vi "Do3.vi"(8 "error in (no error)":errorcluster, 11 "object in":refnum<class "Sub.lvclass">) -> (0 "error out":errorcluster, 2 "Numeric":i32, 3 "object out":refnum<class "Sub.lvclass">)   [LabVIEW 2019, in "Sub.lvclass"]
uses:
  Sub.lvclass
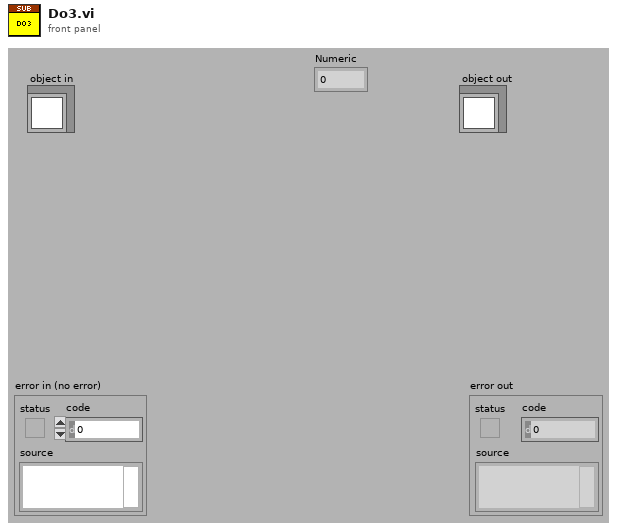
[diagram p1: front panel]
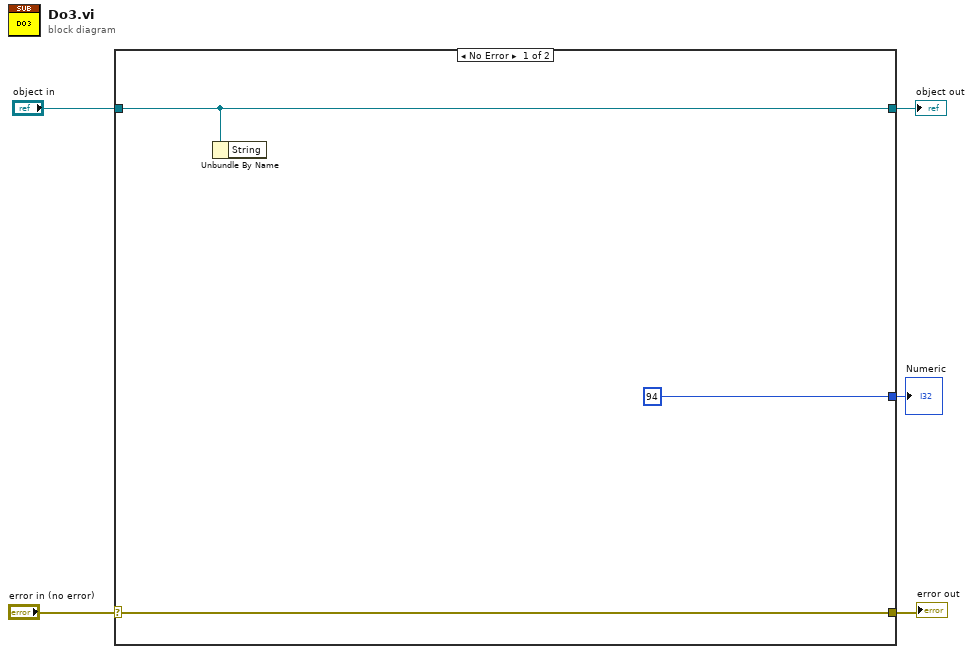
[diagram p0: block diagram]
diagram:
  n1 = case shown="No Error" "error in (no error)" {
    selector: "error in (no error)" -> [w8 w10]
    tunnel: [w8 w10] -> w4
    tunnel: [w7 w9] -> w2
    tunnel: "object in" -> [w7 w9]
    tunnel: [94 _] -> w1
    frame No Error {
      n2 = Unbundle By Name(w7) -> ()  [unwired: 1 out]
    }
    frame Error {
    }
  }
  "error out" <- w4
  "object out" <- w2
  "Numeric" <- w1
